vi "Main.vi"() -> ()   [LabVIEW 2012]
uses:
  Charge Settings TypeDef.ctl
panel:
  in  "Exit":bool
  in  "Tab Control":T1(tab)
  in  "CD max V":dbl caption="Напряжение зарядки, В"
  out "CD Capactor Voltage":dbl[](graph)
  out "CD Current":dbl[](graph)
  in  "Stop C-D":bool
  in  "Start C-D":bool
  in  "Зарядка-разрядка":T2
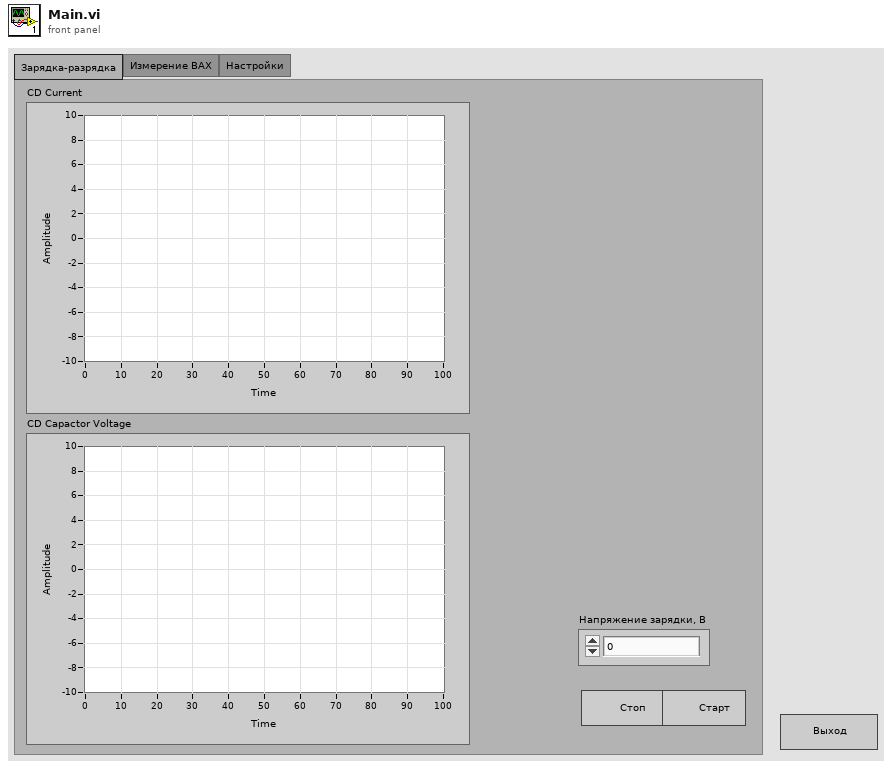
[diagram p1: front panel]
types:
  T1 = enum32{"Зарядка-разрядка", "Измерение ВАХ", "Настройки"}
  T2 = typedef "Charge Settings TypeDef.ctl" = cluster{"Current Input":tag, "Capacitor Voltage Input":tag, "Voltage Output":tag}
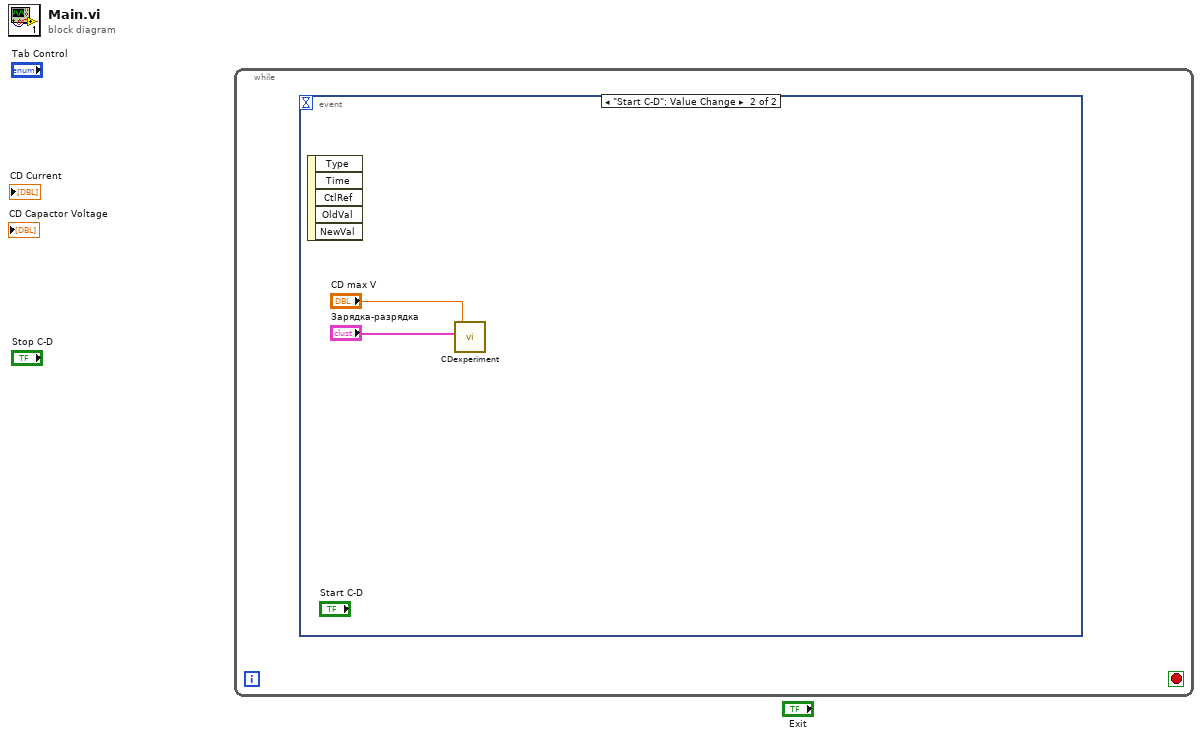
[diagram p0: block diagram]
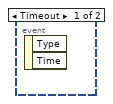
[diagram p2: hidden frame]
diagram:
  n1 = while {
    stop <- _ stop-if-true
    n2 = event shown="[1] \"Start C-D\": Value Change" {
      selector: _ -> [_ _]
      dyn-events: _ -> [_ _]
      timeout: _ -> [_ _]
      event Timeout {
        n3 = event-data() -> ()  [unwired: 1 in, 2 out]
      }
      event "Start C-D": Value Change {
        n4 = event-data() -> ()  [unwired: 1 in, 5 out]
        n5 = call "CDexperiment.vi"("Зарядка-разрядка"="Зарядка-разрядка", "maximum output value"="CD max V") -> ()  [unwired: 3 in, 1 out]
      }
    }
  }
